vi "fotoresistorGOVNOCODE.vi"() -> ()   [LabVIEW 2019]
uses:
  <vilib>/LabVIEW Interface for Arduino/Type Defs/Board Type.ctl
  <vilib>/LabVIEW Interface for Arduino/LabVIEW Interface for Arduino.lvlib
panel:
  in  "Blue Pin":u8
  in  "Green Pin":u8
  in  "Red Pin":u8
  out "Waveform Chart":dbl(graph)
  out "Light Intensity (0 - 100)":dbl(knob) scale=0.0..100.0
  in  "stop":bool
  in  "Photo Cell Pin (0)":u8
  out "error out":errorcluster
  in  "VISA resource":refnum<visa-resource-name>
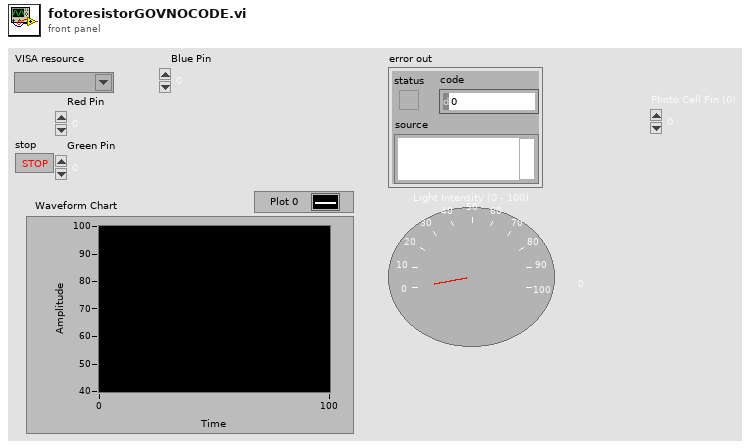
[diagram p1: front panel]
types:
  T1 = typedef "LabVIEW Interface for Arduino.lvlib/Board Type.ctl" = enum16{"Uno", "Dimuelanove w/Atmega 328", "Mega 2560"}
  T2 = typedef "LabVIEW Interface for Arduino.lvlib/Arduino Resource.ctl" = cluster{"VISA resource":refnum<visa-resource-name>, "Board Type":T1, "Connection Type":enum8{"USB / Serial"}, "Bytes Per Packet (15)":u8}
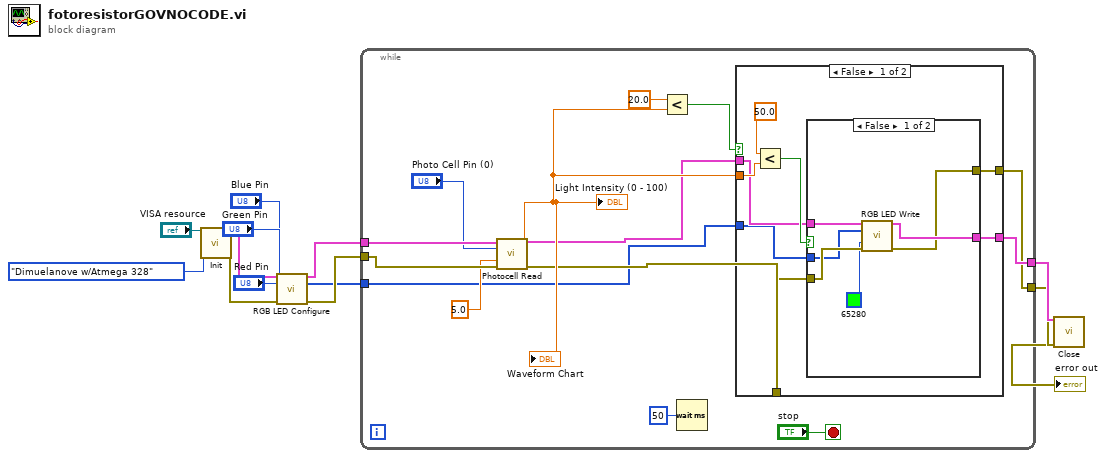
[diagram p0: block diagram]
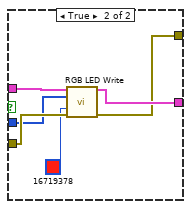
[diagram p2: hidden frame]
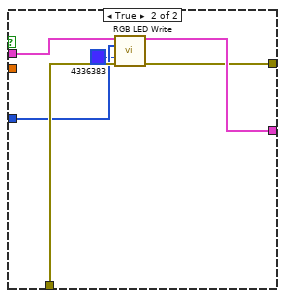
[diagram p3: hidden frame]
diagram:
  n1 = call <vilib>:"Init.vi"("VISA resource"="VISA resource", "Board Type (Uno)"=Board_Type."Dimuelanove w/Atmega 328") -> ("Arduino Resource"=w8:T2, "error out"=w6:errorcluster)  [unwired: 16 in]
  n2 = call <vilib>:"RGB LED Configure.vi"("Arduino Resource"=w8, "Red Pin"="Red Pin", "Green Pin"="Green Pin", "Blue Pin"="Blue Pin", "error in"=w6) -> ("Arduino Resource"=w7:T2, "RGB LED Pins"=w1:u8[], "error out"=w5:errorcluster)  [unwired: 8 in]
  n3 = while {
    tunnel: w7 -> [w27]
    tunnel: w5 -> [w26]
    tunnel: [w19] -> w11
    tunnel: [w18] -> w10
    tunnel: w1 -> [w14]
    stop <- "stop" stop-if-true
    n4 = call <vilib>:"Photocell Read.vi"("Arduino Resource"=w27, "Photo Cell Pin (0)"="Photo Cell Pin (0)", "Vcc (5)"=5.0, "error in"=w26) -> ("Arduino Resource"=w16:T2, "Light Intensity (0 - 100)"=w17:dbl, "error out"=w15:errorcluster)  [unwired: 9 in]
    "Light Intensity (0 - 100)" <- w17
    "Waveform Chart" <- w17
    n5 = Less?(x=20.0, y=w17) -> (x < y?=w20:bool)
    n6 = Wait (ms)(milliseconds to wait=u32 50) -> ()  [unwired: 1 out]
    n7 = case shown="False" w20 {
      tunnel: w16 -> [w32 w53]
      tunnel: w15 -> [w31 w52]
      tunnel: w14 -> [w30 w51]
      tunnel: [w29 w50] -> w19
      tunnel: [w28 w49] -> w18
      tunnel: w17 -> [w34 _]
      frame False {
        n8 = Less?(x=50.0, y=w34) -> (x < y?=w33:bool)
        n9 = case shown="False" w33 {
          tunnel: w32 -> [w41 w47]
          tunnel: w31 -> [w40 w46]
          tunnel: w30 -> [w39 w45]
          tunnel: [w37 w43] -> w29
          tunnel: [w36 w42] -> w28
          frame False {
            n10 = call <vilib>:"RGB LED Write.vi"("Arduino Resource"=w41, "RGB LED Pins"=w39, "Color"=u32 65280, "error in"=w40) -> ("Arduino Resource"=w37:T2, "error out"=w36:errorcluster)  [unwired: 9 in, 1 out]
          }
          frame True {
            n11 = call <vilib>:"RGB LED Write.vi"("Arduino Resource"=w47, "RGB LED Pins"=w45, "Color"=u32 16719378, "error in"=w46) -> ("Arduino Resource"=w43:T2, "error out"=w42:errorcluster)  [unwired: 9 in, 1 out]
          }
        }
      }
      frame True {
        n12 = call <vilib>:"RGB LED Write.vi"("Arduino Resource"=w53, "RGB LED Pins"=w51, "Color"=u32 4336383, "error in"=w52) -> ("Arduino Resource"=w50:T2, "error out"=w49:errorcluster)  [unwired: 9 in, 1 out]
      }
    }
  }
  n13 = call <vilib>:"Close.vi"("Arduino Resource"=w11, "error in"=w10) -> ("error out"=→"error out":errorcluster)  [unwired: 13 in]
